vi "Draw_graph_background.vi"(11 "path":path) -> (3 "Images":picture)   [LabVIEW 2010]
uses:
  gfitsio/gfitsio-read-image-subset-sgl-2d.vi
  <userlib>/gfitsio/gfitsio.lvlib
panel:
  out "Exec Time":u32
  in  "fpixel (1,1)":cluster{"X":i32, "Y":i32}={"X"=1, "Y"=1}
  in  "lpixel (-1,-1: rest)":cluster{"X":i32, "Y":i32}={"X"=-1, "Y"=-1}
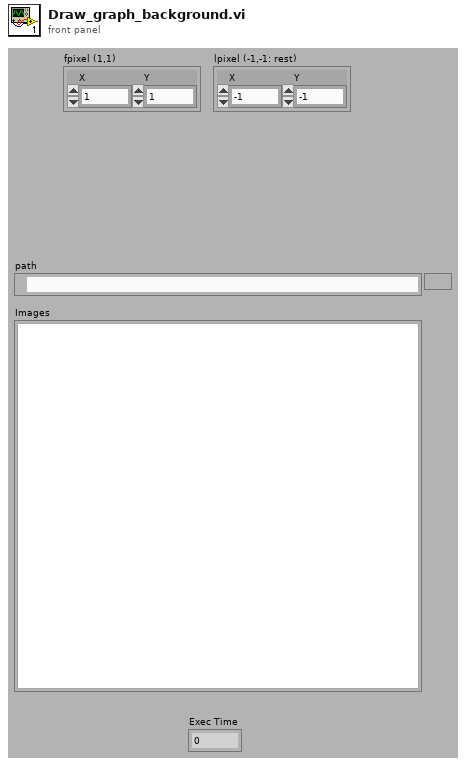
[diagram p1: front panel]
types:
  T1 = typedef "gfitsio.lvlib/gfitsio-refnum.ctl" = refnum<k1>
  T2 = typedef "imagedata.ctl" = cluster{"image type":i32, "image depth":i32, "image":u8[], "mask":u8[], "colors":u32[], "Rectangle":cluster{"left":i16, "top":i16, "right":i16, "bottom":i16}}
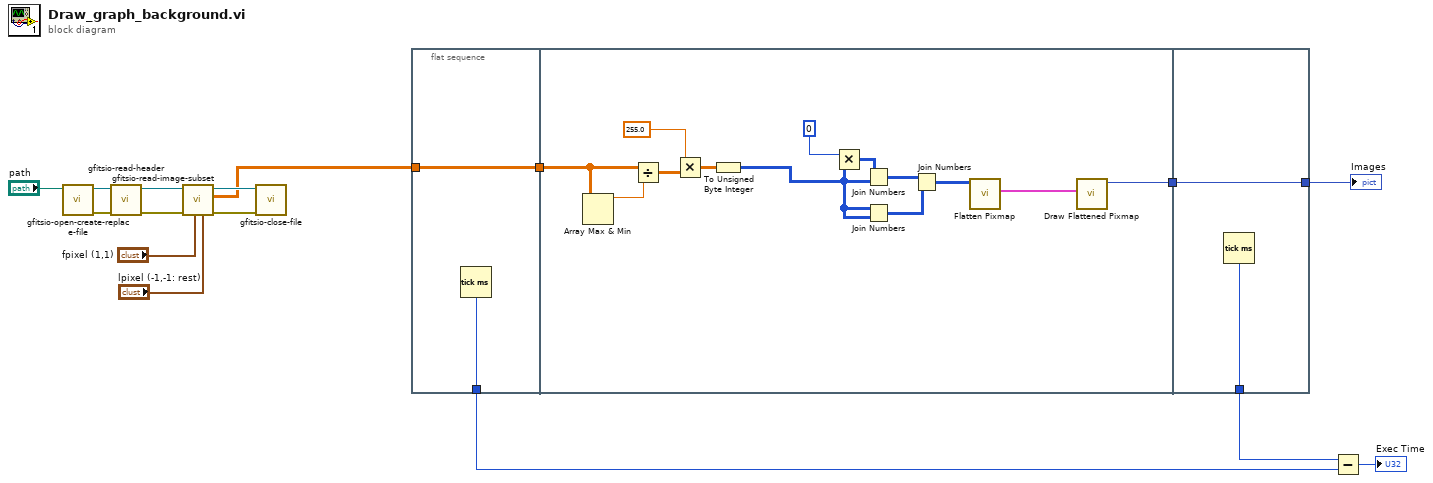
[diagram p0: block diagram]
diagram:
  n1 = call "gfitsio-open-create-replace-file.vi"("file path (dialog if empty)"="path") -> ("error out"=w12:errorcluster, "gfits refnum"=w13:T1)  [unwired: 8 in, 1 out]
  n2 = call "gfitsio-read-header.vi"("error in (no error)"=w12, "gfits refnum"=w13) -> ("error out"=w8:errorcluster, "dup gfits refnum"=w9:T1)  [unwired: 7 in, 1 out]
  n3 = call-poly "gfitsio-read-image-subset.vi"("lpixel (-1,-1: rest)"="lpixel (-1,-1: rest)", "fpixel (1,1)"="fpixel (1,1)", "error in (no error)"=w8, "gfits refnum"=w9) -> ("error out"=w10:errorcluster, "data"=w7:sgl[][], "dup gfits refnum"=w11:T1)  [unwired: 4 in, 1 out]
  n4 = call "gfitsio-close-file.vi"("error in (no error)"=w10, "gfits refnum"=w11) -> ()  [unwired: 8 in, 2 out]
  n5 = flat-sequence {
    tunnel: w7 -> [w18]
    tunnel: [w18] -> w6
    tunnel: [w17] -> w4
    tunnel: w6 -> [w25]
    tunnel: [w19] -> w2
    tunnel: [w33] -> w5
    tunnel: [w32] -> w1
    tunnel: w2 -> [w32]
    frame #0 {
      n6 = Tick Count (ms)() -> (millisecond timer value=w17:u32)
    }
    frame #1 {
      n7 = Array Max & Min(array=w25) -> (max value=w24:sgl)  [unwired: 3 out]
      n8 = Divide(x=w25, y=w24) -> (x/y=w22:sgl[][])
      n9 = Multiply(x=sgl 255.0, y=w22) -> (x*y=w21:sgl[][])
      n10 = To Unsigned Byte Integer(number=w21) -> (unsigned 8bit integer=w20:u8[][])
      n11 = Multiply(x=u8 0, y=w20) -> (x*y=w27:u8[][])
      n12 = Join Numbers(hi=w27, lo=w20) -> ((hi.lo)=w30:u16[][])
      n13 = Join Numbers(hi=w20, lo=w20) -> ((hi.lo)=w29:u16[][])
      n14 = Join Numbers(hi=w30, lo=w29) -> ((hi.lo)=w26:u32[][])
      n15 = call <vilib>:"Flatten Pixmap.vi"("24-bit pixmap"=w26) -> ("image data"=w31:T2)  [unwired: 10 in]
      n16 = call <vilib>:"Draw Flattened Pixmap.vi"("image data"=w31) -> ("new picture"=w19:picture)  [unwired: 8 in]
    }
    frame #2 {
      n17 = Tick Count (ms)() -> (millisecond timer value=w33:u32)
    }
  }
  n18 = Subtract(x=w5, y=w4) -> (x-y=→"Exec Time":u32)
  "Images" <- w1
